vi "Read Config File.vi"(11 "ref in":refnum<k20>) -> (3 "ref out":refnum<k20>)   [LabVIEW 2019]
uses:
  RT Controls/Main Box Config.ctl
  <vilib>/Utility/config.llb/Config Data RefNum.ctl
  <vilib>/Utility/config.llb/Read Key (I32).vi
  <vilib>/Utility/config.llb/Read Key (Boolean).vi
  <vilib>/Utility/config.llb/Read Key (Double).vi
  <vilib>/Utility/config.llb/Read Key (String).vi
  <vilib>/Utility/config.llb/Read Key (U32).vi
  <vilib>/Utility/error.llb/Error Cluster From Error Code.vi
  <vilib>/rvi/errors/niLvFpgaAdjustHostInterfaceError.vi
  <vilib>/rvi/interface/nirviReadWriteControl/nirviReadWriteControl.xnode
  <vilib>/Utility/config.llb/NI_LVConfig.lvlib
  <vilib>/rvi/interface/Simulation/niFpgaSimulationCallBeginRW.vi
  NiFpgaLv.dll
panel:
  in  "LocalAntSecret":string="c3VwcG9ydDphdXh0ZWwyNQ=="
  in  "RemoteAntAddr":string="10.0.1.2"
  in  "LocalAntAddr":string="10.0.1.1"
  out "key errors":errorcluster[](array[cluster])
  out "key":string
  in  "TopAntPort":u16=17309
  in  "TopAntAddr":string="10.0.1.4"
  in  "AntWifi":bool=TRUE
  out "output":T2 {"MainBoxConfig"."Tol" format="%.2f"; "MainBoxConfig"."EncRefDeg" format="%.2f"; "MainBoxConfig"."HomePos" format="%.2f"; "MainBoxConfig"."HSThres" format="%.2f"; "MainBoxConfig"."Coast" format="%.2f"}
  in  "EncCenterTol":u64=5580754
  in  "EncCenterHS":u64=55807545
  in  "EncCenter":u64=68719476735
  in  "AzEncNoError":u16=1025
  out "error out":errorcluster
  out "section exists?":bool
  out "key names":string[](array[string])
  out "file refnum":T3
  in  "MainHostTO":u16=60
  out "config path":path
  in  "MainHostPort":u16=17310
  in  "TopUDPPort":u16=17308
  in  "MainBoxConfig":T1={"WatchdogTim"=600, "DirRevDel"=4, "Coast"=0.5, "HSThres"=5.0, "EncCounts360"=4018143232, "HomePos"=0.0, "EncRefDeg"=0.0, "EncRefCounts"=79895940197, "Tol"=0.5, "CloudEn"=FALSE, "AutoShutEn"=TRUE, "RainTim"=5, "AZTimeout"=120, "AZEncPol"=enum."Positive"} caption="value" {"Tol" format="%.2f"; "EncRefDeg" format="%.2f"; "HomePos" format="%.2f"; "HSThres" format="%.2f"; "Coast" format="%.2f"}
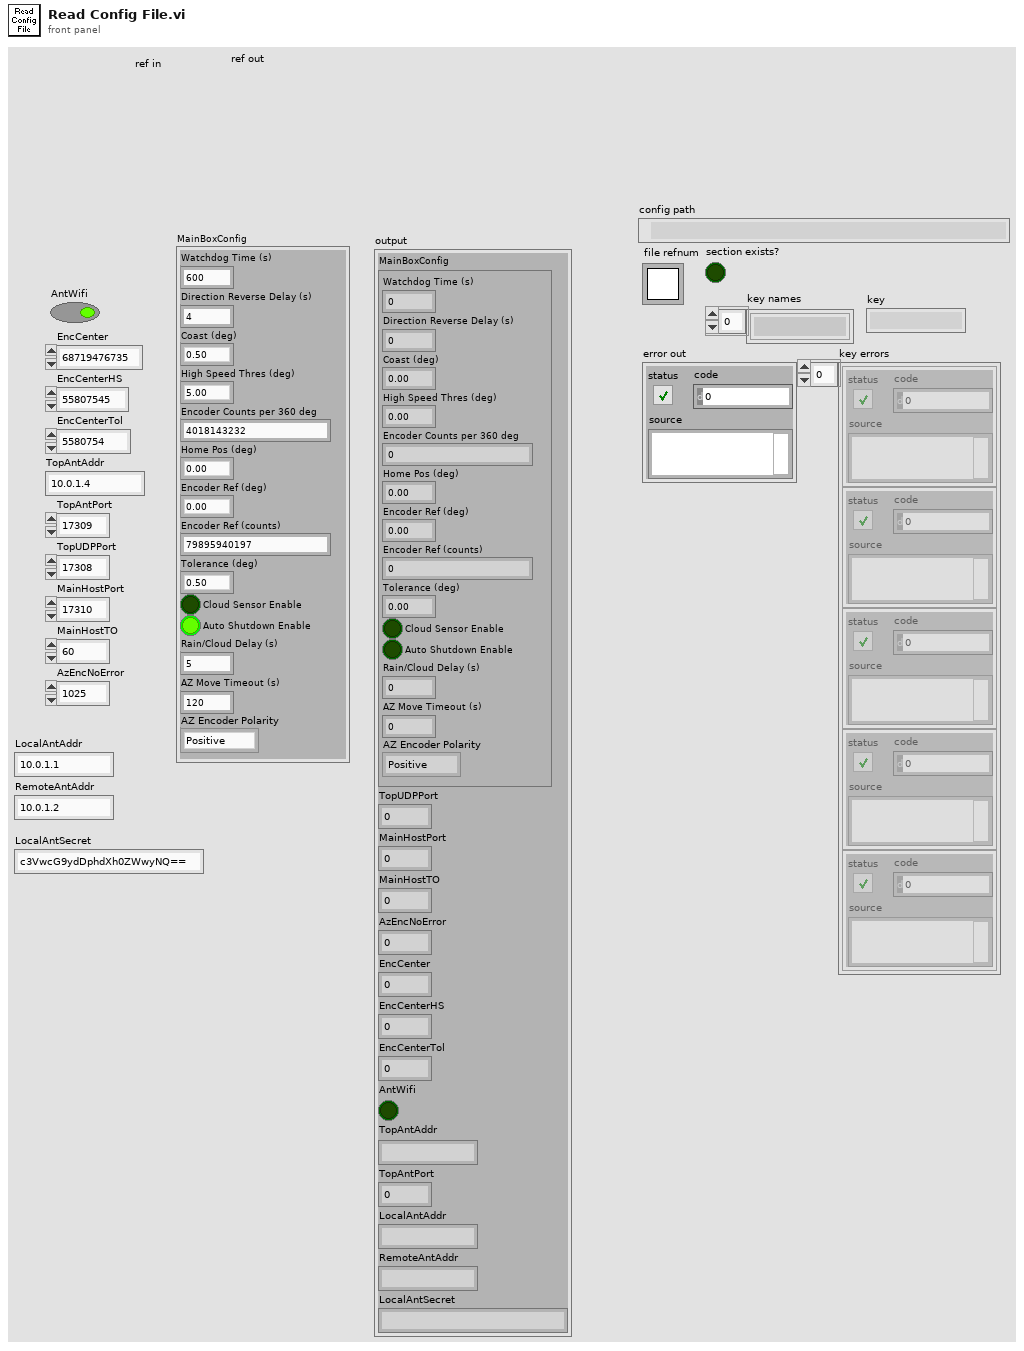
[diagram p1: front panel]
types:
  T1 = typedef "Main Box Config.ctl" = cluster{"WatchdogTim":i32, "DirRevDel":i32, "Coast":dbl, "HSThres":dbl, "EncCounts360":u64, "HomePos":dbl, "EncRefDeg":dbl, "EncRefCounts":u64, "Tol":dbl, "CloudEn":bool, "AutoShutEn":bool, "RainTim":i32, "AZTimeout":i32, "AZEncPol":enum16{"Positive", "Negative"}}
  T2 = cluster{"MainBoxConfig":T1, "TopUDPPort":u16, "MainHostPort":u16, "MainHostTO":u16, "AzEncNoError":u16, "EncCenter":u64, "EncCenterHS":u64, "EncCenterTol":u64, "AntWifi":bool, "TopAntAddr":string, "TopAntPort":u16, "LocalAntAddr":string, "RemoteAntAddr":string, "LocalAntSecret":string}
  T3 = typedef "NI_LVConfig.lvlib/Config Data RefNum.ctl" = refnum<k1>
  T4 = cluster{"io.cloud-enable":bool, "io.encoder-negate":bool, "io.encoder-ref":u64, "io.encoder-step":u64, "io.home-pos":fxp<+/-,32,2>, "sm.az-timeout (ms)":u32, "sm.encoder-no-error":u16, "sm.main-pos-hs-thres":fxp<+/-,32,2>, "sm.main-pos-tol":fxp<+/-,32,2>, "sm.cloud-timeout (ms)":u32, "sm.rev-dly (ms)":u32, "io.encoder-center":u64, "sm-main-center-hs-thres":u64, "sm-main-center-tol":u64}
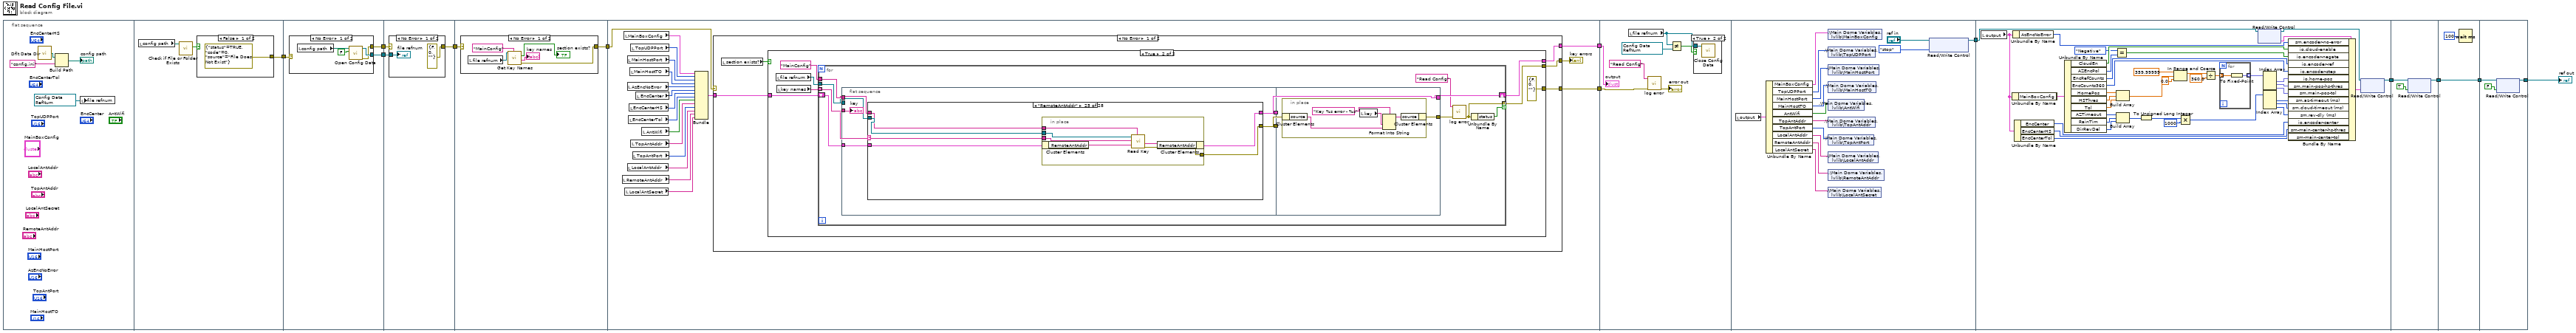
[diagram p0: block diagram]
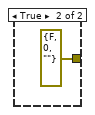
[diagram p2: hidden frame]
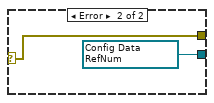
[diagram p3: hidden frame]
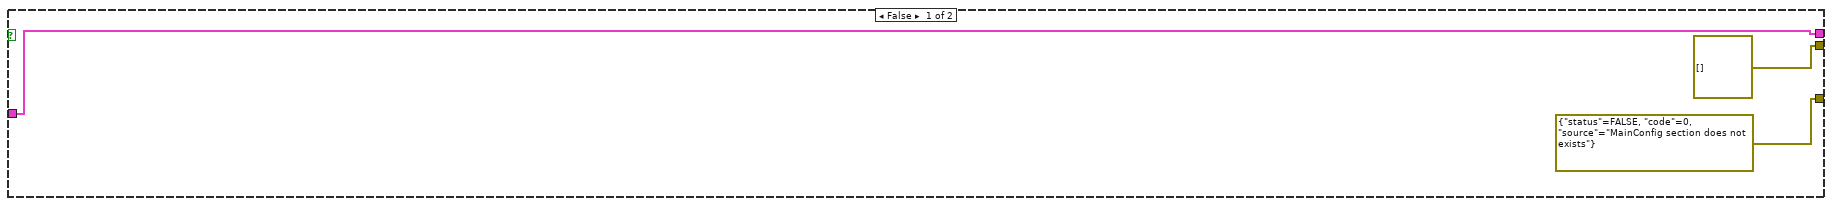
[diagram p6: hidden frame]
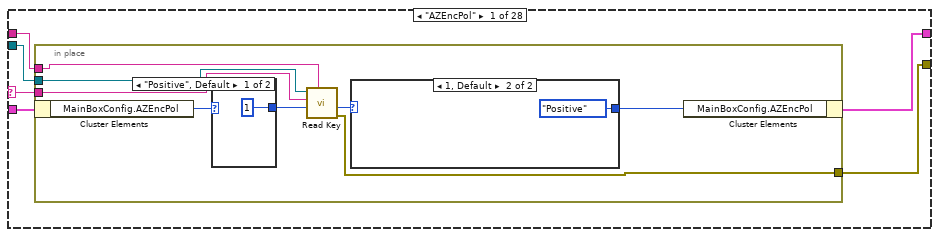
[diagram p7: hidden frame]
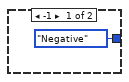
[diagram p8: hidden frame]
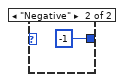
[diagram p9: hidden frame]
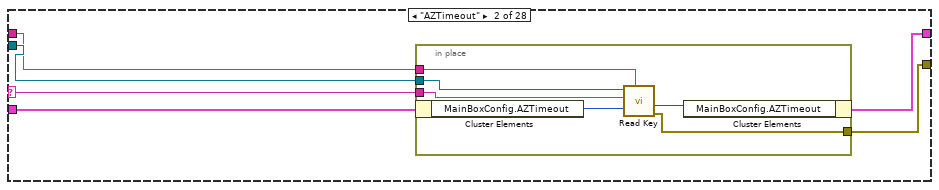
[diagram p10: hidden frame]
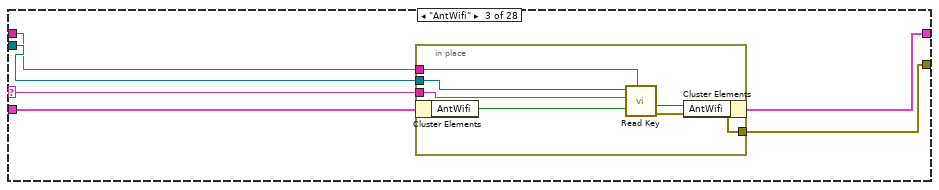
[diagram p11: hidden frame]
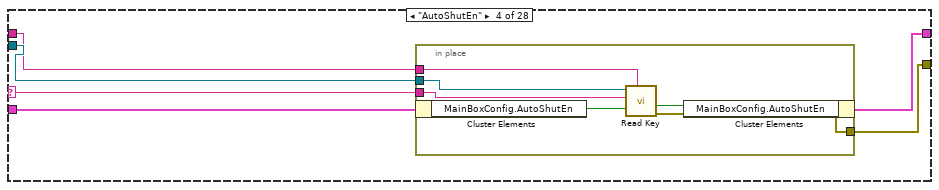
[diagram p12: hidden frame]
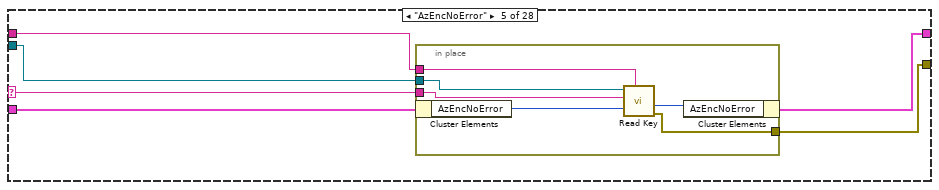
[diagram p13: hidden frame]
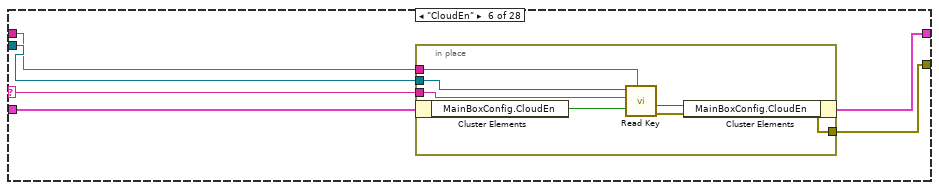
[diagram p14: hidden frame]
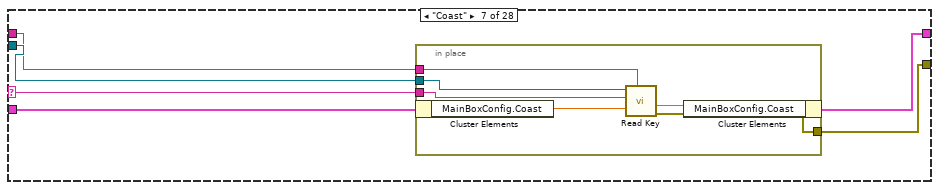
[diagram p15: hidden frame]
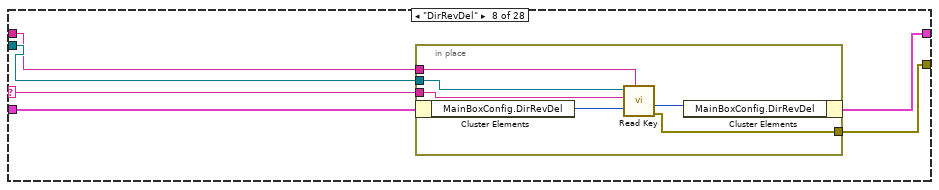
[diagram p16: hidden frame]
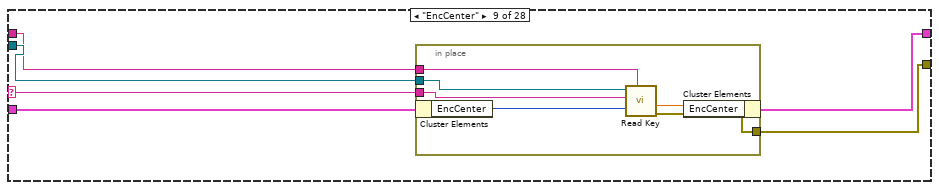
[diagram p17: hidden frame]
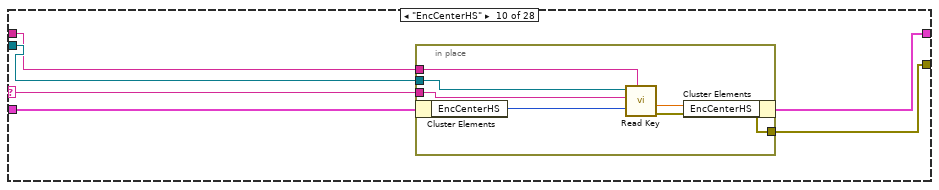
[diagram p18: hidden frame]
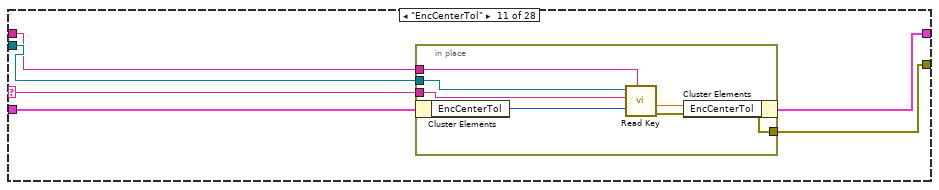
[diagram p19: hidden frame]
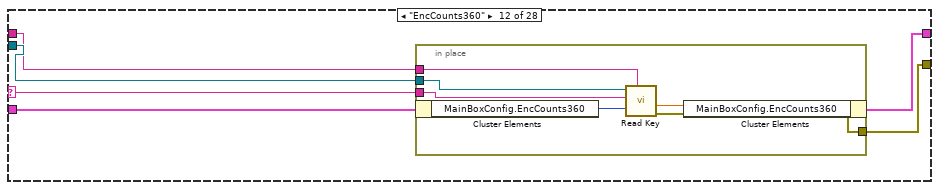
[diagram p20: hidden frame]
diagram:
  n1 = flat-sequence {
    tunnel: [w17] -> w12
    tunnel: w12 -> [w24]
    tunnel: [w23] -> w11
    tunnel: [w22] -> w10
    tunnel: w11 -> [w33]
    tunnel: w10 -> [w32]
    tunnel: [w31] -> w9
    tunnel: w9 -> [w38]
    tunnel: [w37] -> w8
    tunnel: [w63] -> w4
    tunnel: w8 -> [w57]
    tunnel: [w56] -> w3
    tunnel: w4 -> [w441]
    tunnel: w3 -> [w439]
    tunnel: [w450] -> w2
    tunnel: [w498] -> w7
    tunnel: w2 -> [w497]
    tunnel: w7 -> [w504]
    tunnel: [w502] -> w6
    tunnel: w6 -> [w505]
    tunnel: [w505] -> w5
    tunnel: w5 -> [w509]
    tunnel: [w507] -> w1
    frame #0 {
      w13 = T3 refnum items=["config data"] ("file refnum")
      n2 = call <vilib>:"Dflt Data Dir.vi"() -> ("App:Default Data Directory"=w16:path)
      n3 = Build Path(base path=w16, name or relative path="config.ini") -> (appended path=→"config path":path)
      n4 = local write "file refnum"(w13) -> ()
    }
    frame #1 {
      n5 = local read "config path"() -> (w19:path)
      n6 = call <vilib>:"Check if File or Folder Exists.vi"("path"=w19) -> ("file or folder exists?"=w18:bool)  [unwired: 8 in, 2 out]
      n7 = case shown="False" w18 {
        tunnel: [errorcluster {"status"=TRUE, "code"=0, "source"="File Does Not Exist"} ("error constant") errorcluster {"status"=FALSE, "code"=0, "source"=""} ("error constant")] -> w17
        frame False {
        }
        frame True {
        }
      }
    }
    frame #2 {
      n8 = case shown="No Error" w24 {
        selector: w24 -> [_ w29]
        tunnel: [w27 w30] -> w23
        tunnel: [w26 w29] -> w22
        frame No Error {
          n9 = local read "config path"() -> (w28:path)
          n10 = call <vilib>:"Open Config Data.vi"("create file if necessary (T)"=FALSE, "configuration file path"=w28) -> ("error out"=w26:errorcluster, "refnum"=w27:T3)  [unwired: 7 in, 1 out]
        }
        frame Error {
          w30 = T3 refnum items=["config data"] ("refnum")
        }
      }
    }
    frame #3 {
      n11 = case shown="No Error" w32 {
        selector: w32 -> [_ w36]
        tunnel: w33 -> [w35 _]
        tunnel: [errorcluster {"status"=FALSE, "code"=0, "source"=""} ("error IO") w36] -> w31
        frame No Error {
          "file refnum" <- w35
        }
        frame Error {
        }
      }
    }
    frame #4 {
      n12 = case shown="No Error" w38 {
        selector: w38 -> [_ w44]
        tunnel: [w41 w44] -> w37
        frame No Error {
          n13 = local read "file refnum"() -> (w43:T3)
          n14 = call <vilib>:"Get Key Names.vi"("section"="MainConfig", "refnum"=w43) -> ("error out"=w41:errorcluster, "key names"=→"key names":string[], "section exists?"=→"section exists?":bool)  [unwired: 6 in, 1 out]
        }
        frame Error {
        }
      }
    }
    frame #5 {
      n15 = local read "RemoteAntAddr"() -> (w46:string)
      n16 = local read "MainBoxConfig"() -> (w59:T1)
      n17 = local read "LocalAntSecret"() -> (w45:string)
      n18 = local read "MainHostPort"() -> (w61:u16)
      n19 = local read "AzEncNoError"() -> (w55:u16)
      n20 = local read "LocalAntAddr"() -> (w47:string)
      n21 = local read "EncCenterTol"() -> (w52:u64)
      n22 = local read "EncCenterHS"() -> (w53:u64)
      n23 = local read "MainHostTO"() -> (w62:u16)
      n24 = local read "TopUDPPort"() -> (w60:u16)
      n25 = local read "TopAntAddr"() -> (w50:string)
      n26 = local read "TopAntPort"() -> (w49:u16)
      n27 = local read "EncCenter"() -> (w54:u64)
      n28 = local read "AntWifi"() -> (w51:bool)
      n29 = Bundle("MainBoxConfig"=w59, "TopUDPPort"=w60, "MainHostPort"=w61, "MainHostTO"=w62, "AzEncNoError"=w55, "EncCenter"=w54, "EncCenterHS"=w53, "EncCenterTol"=w52, "AntWifi"=w51, "TopAntAddr"=w50, "TopAntPort"=w49, "LocalAntAddr"=w47, "RemoteAntAddr"=w46, "LocalAntSecret"=w45) -> (w58:T2)  [unwired: 1 in]
      n30 = case shown="No Error" w57 {
        selector: w57 -> [_ w436]
        tunnel: [w68 w437] -> w63
        tunnel: w58 -> [w67 w437]
        tunnel: [w65 w436] -> w56
        tunnel: [w64 errorcluster[] []] -> w48
        frame No Error {
          n31 = local read "section exists?"() -> (w66:bool)
          n32 = case shown="True" w66 {
            tunnel: w67 -> [w71 w78]
            tunnel: [w71 w77] -> w68
            tunnel: [errorcluster {"status"=FALSE, "code"=0, "source"="MainConfig section does not exists"} ("error out") errorcluster {"status"=FALSE, "code"=0, "source"=""} ("error out")] -> w65
            tunnel: [errorcluster[] [] w72] -> w64
            frame False {
            }
            frame True {
              n33 = local read "file refnum"() -> (w74:T3)
              n34 = local read "key names"() -> (w76:string[])
              n35 = for {
                tunnel: w76 -> [w89] mode=indexing
                tunnel: w74 -> [w88]
                shift-right: [w86] -> w77
                shift-left: w78 -> [w87]
                tunnel: "MainConfig" ("section") -> [w85]
                tunnel: [w80] -> w72 mode=indexing if=w82
                n36 = flat-sequence {
                  tunnel: w89 -> [w95]
                  tunnel: w88 -> [w94]
                  tunnel: w87 -> [w93]
                  tunnel: w85 -> [w91]
                  tunnel: [w92] -> w84
                  tunnel: [w90] -> w83
                  tunnel: [w430] -> w86
                  tunnel: w84 -> [w430]
                  tunnel: w83 -> [w429]
                  tunnel: [w428] -> w81
                  frame #0 {
                    n37 = case shown="\"RemoteAntAddr\"" w95 {
                      selector: w95 -> [w97 w115 w127 w139 w151 w163 w176 w188 w199 w211 w223 w235 w247 w259 _ w274 w285 w297 w309 w321 w333 w346 w358 w370 w382 w394 w405 w418]
                      tunnel: w94 -> [w99 w117 w129 w141 w152 w165 w177 w189 w201 w213 w225 w237 w249 w261 _ w275 w287 w298 w310 w323 w335 w347 w359 w371 w383 w395 w406 w419]
                      tunnel: w93 -> [w101 w119 w131 w143 w155 w167 w179 w191 w203 w215 w227 w239 w251 w263 w271 w277 w289 w301 w313 w325 w337 w349 w361 w373 w385 w397 w409 w421]
                      tunnel: [w100 w118 w130 w142 w154 w166 w178 w190 w202 w214 w226 w238 w250 w262 w271 w276 w288 w300 w312 w324 w336 w348 w360 w372 w384 w396 w408 w420] -> w92
                      tunnel: w91 -> [w98 w116 w128 w140 w153 w164 w175 w187 w200 w212 w224 w236 w248 w260 _ w273 w286 w299 w311 w322 w334 w345 w357 w369 w381 w393 w407 w417]
                      tunnel: [w96 w114 w126 w138 w150 w162 w174 w186 w198 w210 w222 w234 w246 w258 errorcluster {"status"=FALSE, "code"=0, "source"=""} ("error out") w272 w284 w296 w308 w320 w332 w344 w356 w368 w380 w392 w404 w416] -> w90
                      frame "AZEncPol" {
                        n38 = in-place {
                          in-place-border: w99 -> [w109]
                          in-place-border: w98 -> [w108]
                          in-place-border: w97 -> [w107]
                          in-place-border: [w102] -> w96
                          n39 = in-place-cluster #1(w101) -> ("MainBoxConfig.AZEncPol"=w106:enum16{"Positive", "Negative"})
                          n40 = case shown="\"Positive\", Default" w106 {
                            tunnel: [1 -1] -> w105
                            frame "Positive", Default {
                            }
                            frame "Negative" {
                            }
                          }
                          n41 = call-poly <vilib>:"Read Key.vi"("section"=w108, "default value"=w105, "key"=w107, "refnum"=w109) -> ("error out"=w102:errorcluster, "value"=w104:i32)  [unwired: 4 in, 2 out]
                          n42 = case shown="1, Default" w104 {
                            tunnel: [enum16{"Positive", "Negative"}."Negative" ("AZEncPol") enum16{"Positive", "Negative"}."Positive" ("AZEncPol")] -> w103
                            frame -1 {
                            }
                            frame 1, Default {
                            }
                          }
                          n43 = in-place-cluster #1("MainBoxConfig.AZEncPol"=w103) -> (w100:T2)
                        }
                      }
                      frame "AZTimeout" {
                        n44 = in-place {
                          in-place-border: w117 -> [w125]
                          in-place-border: w116 -> [w122]
                          in-place-border: w115 -> [w121]
                          in-place-border: [w120] -> w114
                          n45 = in-place-cluster #2(w119) -> ("MainBoxConfig.AZTimeout"=w124:i32)
                          n46 = call-poly <vilib>:"Read Key.vi"("section"=w122, "default value"=w124, "key"=w121, "refnum"=w125) -> ("error out"=w120:errorcluster, "value"=w123:i32)  [unwired: 4 in, 2 out]
                          n47 = in-place-cluster #2("MainBoxConfig.AZTimeout"=w123) -> (w118:T2)
                        }
                      }
                      frame "AntWifi" {
                        n48 = in-place {
                          in-place-border: w129 -> [w137]
                          in-place-border: w128 -> [w134]
                          in-place-border: w127 -> [w133]
                          in-place-border: [w132] -> w126
                          n49 = in-place-cluster #3(w131) -> ("AntWifi"=w136:bool)
                          n50 = call-poly <vilib>:"Read Key.vi"("section"=w134, "default value"=w136, "key"=w133, "refnum"=w137) -> ("error out"=w132:errorcluster, "value"=w135:bool)  [unwired: 4 in, 2 out]
                          n51 = in-place-cluster #3("AntWifi"=w135) -> (w130:T2)
                        }
                      }
                      frame "AutoShutEn" {
                        n52 = in-place {
                          in-place-border: w141 -> [w149]
                          in-place-border: w140 -> [w146]
                          in-place-border: w139 -> [w145]
                          in-place-border: [w144] -> w138
                          n53 = in-place-cluster #4(w143) -> ("MainBoxConfig.AutoShutEn"=w148:bool)
                          n54 = call-poly <vilib>:"Read Key.vi"("section"=w146, "default value"=w148, "key"=w145, "refnum"=w149) -> ("error out"=w144:errorcluster, "value"=w147:bool)  [unwired: 4 in, 2 out]
                          n55 = in-place-cluster #4("MainBoxConfig.AutoShutEn"=w147) -> (w142:T2)
                        }
                      }
                      frame "AzEncNoError" {
                        n56 = in-place {
                          in-place-border: w152 -> [w161]
                          in-place-border: w151 -> [w158]
                          in-place-border: w153 -> [w157]
                          in-place-border: [w156] -> w150
                          n57 = in-place-cluster #5(w155) -> ("AzEncNoError"=w160:u16)
                          n58 = call-poly <vilib>:"Read Key.vi"("section"=w157, "default value"=w160, "key"=w158, "refnum"=w161) -> ("error out"=w156:errorcluster, "value"=w159:i32)  [unwired: 4 in, 2 out]
                          n59 = in-place-cluster #5("AzEncNoError"=w159) -> (w154:T2)
                        }
                      }
                      frame "CloudEn" {
                        n60 = in-place {
                          in-place-border: w165 -> [w173]
                          in-place-border: w164 -> [w170]
                          in-place-border: w163 -> [w169]
                          in-place-border: [w168] -> w162
                          n61 = in-place-cluster #6(w167) -> ("MainBoxConfig.CloudEn"=w172:bool)
                          n62 = call-poly <vilib>:"Read Key.vi"("section"=w170, "default value"=w172, "key"=w169, "refnum"=w173) -> ("error out"=w168:errorcluster, "value"=w171:bool)  [unwired: 4 in, 2 out]
                          n63 = in-place-cluster #6("MainBoxConfig.CloudEn"=w171) -> (w166:T2)
                        }
                      }
                      frame "Coast" {
                        n64 = in-place {
                          in-place-border: w177 -> [w185]
                          in-place-border: w176 -> [w182]
                          in-place-border: w175 -> [w181]
                          in-place-border: [w180] -> w174
                          n65 = in-place-cluster #7(w179) -> ("MainBoxConfig.Coast"=w184:dbl)
                          n66 = call-poly <vilib>:"Read Key.vi"("section"=w181, "default value"=w184, "key"=w182, "refnum"=w185) -> ("error out"=w180:errorcluster, "value"=w183:dbl)  [unwired: 4 in, 2 out]
                          n67 = in-place-cluster #7("MainBoxConfig.Coast"=w183) -> (w178:T2)
                        }
                      }
                      frame "DirRevDel" {
                        n68 = in-place {
                          in-place-border: w189 -> [w197]
                          in-place-border: w188 -> [w194]
                          in-place-border: w187 -> [w193]
                          in-place-border: [w192] -> w186
                          n69 = in-place-cluster #8(w191) -> ("MainBoxConfig.DirRevDel"=w196:i32)
                          n70 = call-poly <vilib>:"Read Key.vi"("section"=w193, "default value"=w196, "key"=w194, "refnum"=w197) -> ("error out"=w192:errorcluster, "value"=w195:i32)  [unwired: 4 in, 2 out]
                          n71 = in-place-cluster #8("MainBoxConfig.DirRevDel"=w195) -> (w190:T2)
                        }
                      }
                      frame "EncCenter" {
                        n72 = in-place {
                          in-place-border: w201 -> [w209]
                          in-place-border: w200 -> [w206]
                          in-place-border: w199 -> [w205]
                          in-place-border: [w204] -> w198
                          n73 = in-place-cluster #9(w203) -> ("EncCenter"=w208:u64)
                          n74 = call-poly <vilib>:"Read Key.vi"("section"=w206, "default value"=w208, "key"=w205, "refnum"=w209) -> ("error out"=w204:errorcluster, "value"=w207:dbl)  [unwired: 4 in, 2 out]
                          n75 = in-place-cluster #9("EncCenter"=w207) -> (w202:T2)
                        }
                      }
                      frame "EncCenterHS" {
                        n76 = in-place {
                          in-place-border: w213 -> [w221]
                          in-place-border: w212 -> [w218]
                          in-place-border: w211 -> [w217]
                          in-place-border: [w216] -> w210
                          n77 = in-place-cluster #10(w215) -> ("EncCenterHS"=w220:u64)
                          n78 = call-poly <vilib>:"Read Key.vi"("section"=w218, "default value"=w220, "key"=w217, "refnum"=w221) -> ("error out"=w216:errorcluster, "value"=w219:dbl)  [unwired: 4 in, 2 out]
                          n79 = in-place-cluster #10("EncCenterHS"=w219) -> (w214:T2)
                        }
                      }
                      frame "EncCenterTol" {
                        n80 = in-place {
                          in-place-border: w225 -> [w233]
                          in-place-border: w224 -> [w230]
                          in-place-border: w223 -> [w229]
                          in-place-border: [w228] -> w222
                          n81 = in-place-cluster #11(w227) -> ("EncCenterTol"=w232:u64)
                          n82 = call-poly <vilib>:"Read Key.vi"("section"=w230, "default value"=w232, "key"=w229, "refnum"=w233) -> ("error out"=w228:errorcluster, "value"=w231:dbl)  [unwired: 4 in, 2 out]
                          n83 = in-place-cluster #11("EncCenterTol"=w231) -> (w226:T2)
                        }
                      }
                      frame "EncCounts360" {
                        n84 = in-place {
                          in-place-border: w237 -> [w245]
                          in-place-border: w236 -> [w242]
                          in-place-border: w235 -> [w241]
                          in-place-border: [w240] -> w234
                          n85 = in-place-cluster #12(w239) -> ("MainBoxConfig.EncCounts360"=w244:u64)
                          n86 = call-poly <vilib>:"Read Key.vi"("section"=w242, "default value"=w244, "key"=w241, "refnum"=w245) -> ("error out"=w240:errorcluster, "value"=w243:dbl)  [unwired: 4 in, 2 out]
                          n87 = in-place-cluster #12("MainBoxConfig.EncCounts360"=w243) -> (w238:T2)
                        }
                      }
                      frame "EncRefCounts" {
                        n88 = in-place {
                          in-place-border: w249 -> [w257]
                          in-place-border: w248 -> [w254]
                          in-place-border: w247 -> [w253]
                          in-place-border: [w252] -> w246
                          n89 = in-place-cluster #13(w251) -> ("MainBoxConfig.EncRefCounts"=w256:u64)
                          n90 = call-poly <vilib>:"Read Key.vi"("section"=w254, "default value"=w256, "key"=w253, "refnum"=w257) -> ("error out"=w252:errorcluster, "value"=w255:dbl)  [unwired: 4 in, 2 out]
                          n91 = in-place-cluster #13("MainBoxConfig.EncRefCounts"=w255) -> (w250:T2)
                        }
                      }
                      frame "EncRefDeg" {
                        n92 = in-place {
                          in-place-border: w261 -> [w269]
                          in-place-border: w260 -> [w266]
                          in-place-border: w259 -> [w265]
                          in-place-border: [w264] -> w258
                          n93 = in-place-cluster #14(w263) -> ("MainBoxConfig.EncRefDeg"=w268:dbl)
                          n94 = call-poly <vilib>:"Read Key.vi"("section"=w266, "default value"=w268, "key"=w265, "refnum"=w269) -> ("error out"=w264:errorcluster, "value"=w267:dbl)  [unwired: 4 in, 2 out]
                          n95 = in-place-cluster #14("MainBoxConfig.EncRefDeg"=w267) -> (w262:T2)
                        }
                      }
                      frame "False", Default {
                      }
                      frame "HSThres" {
                        n96 = in-place {
                          in-place-border: w275 -> [w283]
                          in-place-border: w274 -> [w280]
                          in-place-border: w273 -> [w279]
                          in-place-border: [w278] -> w272
                          n97 = in-place-cluster #15(w277) -> ("MainBoxConfig.HSThres"=w282:dbl)
                          n98 = call-poly <vilib>:"Read Key.vi"("section"=w279, "default value"=w282, "key"=w280, "refnum"=w283) -> ("error out"=w278:errorcluster, "value"=w281:dbl)  [unwired: 4 in, 2 out]
                          n99 = in-place-cluster #15("MainBoxConfig.HSThres"=w281) -> (w276:T2)
                        }
                      }
                      frame "HomePos" {
                        n100 = in-place {
                          in-place-border: w287 -> [w295]
                          in-place-border: w286 -> [w292]
                          in-place-border: w285 -> [w291]
                          in-place-border: [w290] -> w284
                          n101 = in-place-cluster #16(w289) -> ("MainBoxConfig.HomePos"=w294:dbl)
                          n102 = call-poly <vilib>:"Read Key.vi"("section"=w292, "default value"=w294, "key"=w291, "refnum"=w295) -> ("error out"=w290:errorcluster, "value"=w293:dbl)  [unwired: 4 in, 2 out]
                          n103 = in-place-cluster #16("MainBoxConfig.HomePos"=w293) -> (w288:T2)
                        }
                      }
                      frame "MainHostPort" {
                        n104 = in-place {
                          in-place-border: w298 -> [w307]
                          in-place-border: w297 -> [w304]
                          in-place-border: w299 -> [w303]
                          in-place-border: [w302] -> w296
                          n105 = in-place-cluster #17(w301) -> ("MainHostPort"=w306:u16)
                          n106 = call-poly <vilib>:"Read Key.vi"("section"=w303, "default value"=w306, "key"=w304, "refnum"=w307) -> ("error out"=w302:errorcluster, "value"=w305:i32)  [unwired: 4 in, 2 out]
                          n107 = in-place-cluster #17("MainHostPort"=w305) -> (w300:T2)
                        }
                      }
                      frame "MainHostTO" {
                        n108 = in-place {
                          in-place-border: w310 -> [w319]
                          in-place-border: w309 -> [w316]
                          in-place-border: w311 -> [w315]
                          in-place-border: [w314] -> w308
                          n109 = in-place-cluster #18(w313) -> ("MainHostTO"=w318:u16)
                          n110 = call-poly <vilib>:"Read Key.vi"("section"=w315, "default value"=w318, "key"=w316, "refnum"=w319) -> ("error out"=w314:errorcluster, "value"=w317:i32)  [unwired: 4 in, 2 out]
                          n111 = in-place-cluster #18("MainHostTO"=w317) -> (w312:T2)
                        }
                      }
                      frame "RainTim" {
                        n112 = in-place {
                          in-place-border: w323 -> [w331]
                          in-place-border: w322 -> [w328]
                          in-place-border: w321 -> [w327]
                          in-place-border: [w326] -> w320
                          n113 = in-place-cluster #19(w325) -> ("MainBoxConfig.RainTim"=w330:i32)
                          n114 = call-poly <vilib>:"Read Key.vi"("section"=w328, "default value"=w330, "key"=w327, "refnum"=w331) -> ("error out"=w326:errorcluster, "value"=w329:i32)  [unwired: 4 in, 2 out]
                          n115 = in-place-cluster #19("MainBoxConfig.RainTim"=w329) -> (w324:T2)
                        }
                      }
                      frame "Tol" {
                        n116 = in-place {
                          in-place-border: w335 -> [w343]
                          in-place-border: w334 -> [w340]
                          in-place-border: w333 -> [w339]
                          in-place-border: [w338] -> w332
                          n117 = in-place-cluster #20(w337) -> ("MainBoxConfig.Tol"=w342:dbl)
                          n118 = call-poly <vilib>:"Read Key.vi"("section"=w340, "default value"=w342, "key"=w339, "refnum"=w343) -> ("error out"=w338:errorcluster, "value"=w341:dbl)  [unwired: 4 in, 2 out]
                          n119 = in-place-cluster #20("MainBoxConfig.Tol"=w341) -> (w336:T2)
                        }
                      }
                      frame "TopAntAddr" {
                        n120 = in-place {
                          in-place-border: w347 -> [w355]
                          in-place-border: w346 -> [w352]
                          in-place-border: w345 -> [w351]
                          in-place-border: [w350] -> w344
                          n121 = in-place-cluster #21(w349) -> ("TopAntAddr"=w354:string)
                          n122 = call-poly <vilib>:"Read Key.vi"("section"=w351, "default value"=w354, "key"=w352, "refnum"=w355) -> ("error out"=w350:errorcluster, "value"=w353:string)  [unwired: 4 in, 2 out]
                          n123 = in-place-cluster #21("TopAntAddr"=w353) -> (w348:T2)
                        }
                      }
                      frame "LocalAntAddr" {
                        n124 = in-place {
                          in-place-border: w359 -> [w367]
                          in-place-border: w358 -> [w364]
                          in-place-border: w357 -> [w363]
                          in-place-border: [w362] -> w356
                          n125 = in-place-cluster #22(w361) -> ("LocalAntAddr"=w366:string)
                          n126 = call-poly <vilib>:"Read Key.vi"("section"=w363, "default value"=w366, "key"=w364, "refnum"=w367) -> ("error out"=w362:errorcluster, "value"=w365:string)  [unwired: 4 in, 2 out]
                          n127 = in-place-cluster #22("LocalAntAddr"=w365) -> (w360:T2)
                        }
                      }
                      frame "LocalAntSecret" {
                        n128 = in-place {
                          in-place-border: w371 -> [w379]
                          in-place-border: w370 -> [w376]
                          in-place-border: w369 -> [w375]
                          in-place-border: [w374] -> w368
                          n129 = in-place-cluster #23(w373) -> ("LocalAntSecret"=w378:string)
                          n130 = call-poly <vilib>:"Read Key.vi"("section"=w375, "default value"=w378, "key"=w376, "refnum"=w379) -> ("error out"=w374:errorcluster, "value"=w377:string)  [unwired: 4 in, 2 out]
                          n131 = in-place-cluster #23("LocalAntSecret"=w377) -> (w372:T2)
                        }
                      }
                      frame "RemoteAntAddr" {
                        n132 = in-place {
                          in-place-border: w383 -> [w391]
                          in-place-border: w382 -> [w388]
                          in-place-border: w381 -> [w387]
                          in-place-border: [w386] -> w380
                          n133 = in-place-cluster #24(w385) -> ("RemoteAntAddr"=w390:string)
                          n134 = call-poly <vilib>:"Read Key.vi"("section"=w387, "default value"=w390, "key"=w388, "refnum"=w391) -> ("error out"=w386:errorcluster, "value"=w389:string)  [unwired: 4 in, 2 out]
                          n135 = in-place-cluster #24("RemoteAntAddr"=w389) -> (w384:T2)
                        }
                      }
                      frame "TopAntPort" {
                        n136 = in-place {
                          in-place-border: w395 -> [w403]
                          in-place-border: w394 -> [w400]
                          in-place-border: w393 -> [w399]
                          in-place-border: [w398] -> w392
                          n137 = in-place-cluster #25(w397) -> ("TopAntPort"=w402:u16)
                          n138 = call-poly <vilib>:"Read Key.vi"("section"=w399, "default value"=w402, "key"=w400, "refnum"=w403) -> ("error out"=w398:errorcluster, "value"=w401:u32)  [unwired: 4 in, 2 out]
                          n139 = in-place-cluster #25("TopAntPort"=w401) -> (w396:T2)
                        }
                      }
                      frame "TopUDPPort" {
                        n140 = in-place {
                          in-place-border: w406 -> [w415]
                          in-place-border: w405 -> [w412]
                          in-place-border: w407 -> [w411]
                          in-place-border: [w410] -> w404
                          n141 = in-place-cluster #26(w409) -> ("TopUDPPort"=w414:u16)
                          n142 = call-poly <vilib>:"Read Key.vi"("section"=w411, "default value"=w414, "key"=w412, "refnum"=w415) -> ("error out"=w410:errorcluster, "value"=w413:i32)  [unwired: 4 in, 2 out]
                          n143 = in-place-cluster #26("TopUDPPort"=w413) -> (w408:T2)
                        }
                      }
                      frame "WatchdogTim" {
                        n144 = in-place {
                          in-place-border: w419 -> [w427]
                          in-place-border: w418 -> [w424]
                          in-place-border: w417 -> [w423]
                          in-place-border: [w422] -> w416
                          n145 = in-place-cluster #27(w421) -> ("MainBoxConfig.WatchdogTim"=w426:i32)
                          n146 = call-poly <vilib>:"Read Key.vi"("section"=w423, "default value"=w426, "key"=w424, "refnum"=w427) -> ("error out"=w422:errorcluster, "value"=w425:i32)  [unwired: 4 in, 2 out]
                          n147 = in-place-cluster #27("MainBoxConfig.WatchdogTim"=w425) -> (w420:T2)
                        }
                      }
                    }
                    "key" <- w95
                  }
                  frame #1 {
                    n148 = in-place {
                      n149 = in-place-cluster #28(w429) -> ("source"=w433:string)
                      n150 = local read "key"() -> (w431:string)
                      n151 = Format Into String(format string="Key %s error - %s", w431, w433) -> (resulting string=w432:string)  [unwired: 2 in, 1 out]
                      n152 = in-place-cluster #28("source"=w432) -> (w428:errorcluster)
                    }
                  }
                }
                n153 = call "log error.vi"("error in"=w81, "message"="Read Config") -> ("error out"=w80:errorcluster)  [unwired: 9 in]
                n154 = Unbundle By Name(w80) -> ("status"=w82:bool)
              }
            }
          }
        }
        frame Error {
        }
      }
      "key errors" <- w48
    }
    frame #6 {
      w442 = T3 refnum items=["config data"] ("y")
      n155 = local read "file refnum"() -> (w444:T3)
      n156 = call "log error.vi"("error in"=w439, "message"="Read Config") -> ("error out"=→"error out":errorcluster)  [unwired: 9 in]
      n157 = Not Equal?(x=w444, y=w442) -> (x != y?=w443:bool)
      n158 = case shown="True" w443 {
        tunnel: w444 -> [_ w445]
        frame False {
        }
        frame True {
          n159 = call <vilib>:"Close Config Data.vi"("refnum"=w445) -> ()  [unwired: 9 in, 2 out]
        }
      }
      "output" <- w441
    }
    frame #7 {
      n160 = local read "output"() -> (w455:T2)
      n161 = Unbundle By Name(w455) -> ("MainBoxConfig"=w456:T1, "TopUDPPort"=w459:u16, "MainHostPort"=w458:u16, "MainHostTO"=w457:u16, "AntWifi"=w454:bool, "TopAntAddr"=w453:string, "TopAntPort"=w452:u16, "LocalAntAddr"=w448:string, "RemoteAntAddr"=w447:string, "LocalAntSecret"=w446:string)
      n162 = shared-variable ".\\Main Dome Variables.lvlib\\MainBoxConfig"(w456) -> ()  [unwired: 1 in, 1 out]
      n163 = shared-variable ".\\Main Dome Variables.lvlib\\TopUDPPort"(w459) -> ()  [unwired: 1 in, 1 out]
      n164 = shared-variable ".\\Main Dome Variables.lvlib\\MainHostPort"(w458) -> ()  [unwired: 1 in, 1 out]
      n165 = shared-variable ".\\Main Dome Variables.lvlib\\MainHostTO"(w457) -> ()  [unwired: 1 in, 1 out]
      n166 = shared-variable ".\\Main Dome Variables.lvlib\\AntWifi"(w454) -> ()  [unwired: 1 in, 1 out]
      n167 = shared-variable ".\\Main Dome Variables.lvlib\\TopAntAddr"(w453) -> ()  [unwired: 1 in, 1 out]
      n168 = shared-variable ".\\Main Dome Variables.lvlib\\TopAntPort"(w452) -> ()  [unwired: 1 in, 1 out]
      n169 = shared-variable ".\\Main Dome Variables.lvlib\\LocalAntAddr"(w448) -> ()  [unwired: 1 in, 1 out]
      n170 = shared-variable ".\\Main Dome Variables.lvlib\\RemoteAntAddr"(w447) -> ()  [unwired: 1 in, 1 out]
      n171 = shared-variable ".\\Main Dome Variables.lvlib\\LocalAntSecret"(w446) -> ()  [unwired: 1 in, 1 out]
      n172 = xnode "Read/Write Control"("FPGA VI Reference In"="ref in", "mode request"=enum16{"stop", "home", "position", "center"}."stop") -> ("FPGA VI Reference Out"=w450:refnum<k20>)  [unwired: 1 in, 1 out]
    }
    frame #8 {
      n173 = local read "output"() -> (w463:T2)
      n174 = Unbundle By Name(w463) -> ("MainBoxConfig"=w477:T1)
      n175 = Unbundle By Name(w463) -> ("AzEncNoError"=w464:u16)
      n176 = Unbundle By Name(w463) -> ("EncCenter"=w462:u64, "EncCenterHS"=w461:u64, "EncCenterTol"=w460:u64)
      n177 = Unbundle By Name(w477) -> ("CloudEn"=w472:bool, "AZEncPol"=w473:enum16{"Positive", "Negative"}, "EncRefCounts"=w475:u64, "EncCounts360"=w476:u64, "HomePos"=w478:dbl, "HSThres"=w479:dbl, "Tol"=w480:dbl, "AZTimeout"=w488:i32, "RainTim"=w489:i32, "DirRevDel"=w490:i32)
      n178 = Equal?(x=enum16{"Positive", "Negative"}."Negative", y=w473) -> (x = y?=w474:bool)
      n179 = Build Array(w478, w479, w480) -> (w481:dbl[])
      n180 = Build Array(w488, w489, w490) -> (w491:i32[])
      n181 = To Unsigned Long Integer(number=w491) -> (unsigned 32bit integer=w492:u32[])
      n182 = In Range and Coerce(upper limit=359.99999, x=w481, lower limit=0.0 ("upper limit")) -> (coerced(x)=w482:dbl[])  [unwired: 1 out]
      n183 = Multiply(x=w492, y=u32 1000 ("sm.rev-dly (ms)")) -> (x*y=w493:u32[])
      n184 = Divide(x=w482, y=360.0 ("upper limit")) -> (x/y=w483:dbl[])
      n185 = for {
        tunnel: w483 -> [w501] mode=indexing
        tunnel: [w500] -> w484 mode=indexing
        n186 = To Fixed-Point(number=w501) -> (fixed-point=w500:fxp<+/-,32,2>)  [unwired: 1 in]
      }
      n187 = xnode "Read/Write Control"("FPGA VI Reference In"=w497) -> ("FPGA VI Reference Out"=w499:refnum<k20>, "config"=w466:T4)  [unwired: 1 in, 1 out]
      n188 = Index Array(array=w484) -> (element #1=w485:fxp<+/-,32,2>, element #2=w486:fxp<+/-,32,2>, element #3=w487:fxp<+/-,32,2>)  [unwired: 3 in]
      n189 = Index Array(array=w493) -> (element #1=w494:u32, element #2=w495:u32, element #3=w496:u32)  [unwired: 3 in]
      n190 = Bundle By Name(cluster=w466, "sm.encoder-no-error"=w464, "io.cloud-enable"=w472, "io.encoder-negate"=w474, "io.encoder-ref"=w475, "io.encoder-step"=w476, "io.home-pos"=w485, "sm.main-pos-hs-thres"=w486, "sm.main-pos-tol"=w487, "sm.az-timeout (ms)"=w494, "sm.cloud-timeout (ms)"=w495, "sm.rev-dly (ms)"=w496, "io.encoder-center"=w462, "sm-main-center-hs-thres"=w461, "sm-main-center-tol"=w460) -> (w465:T4)
      n191 = xnode "Read/Write Control"("FPGA VI Reference In"=w499, "config"=w465) -> ("FPGA VI Reference Out"=w498:refnum<k20>)  [unwired: 1 in, 1 out]
    }
    frame #9 {
      n192 = xnode "Read/Write Control"("FPGA VI Reference In"=w504, "reset"=TRUE) -> ("FPGA VI Reference Out"=w502:refnum<k20>)  [unwired: 1 in, 1 out]
    }
    frame #10 {
      n193 = Wait (ms)(milliseconds to wait=u32 100) -> ()  [unwired: 1 out]
    }
    frame #11 {
      n194 = xnode "Read/Write Control"("FPGA VI Reference In"=w509, "reset"=FALSE) -> ("FPGA VI Reference Out"=w507:refnum<k20>)  [unwired: 1 in, 1 out]
    }
  }
  "ref out" <- w1
